vi "compute_average_movie.vi"(8 "error in (no error)":errorcluster, 10 "movies":refnum<class "ImageCollection.lvclass">[](array[class])) -> (0 "error out":errorcluster, 2 "average movie":refnum<class "ImageCollection.lvclass">)   [LabVIEW 2010, in "ImageCollection.lvclass"]
uses:
  ImageCollection.lvclass
  Image/Image/Image.lvclass
  add_mode_enum.ctl
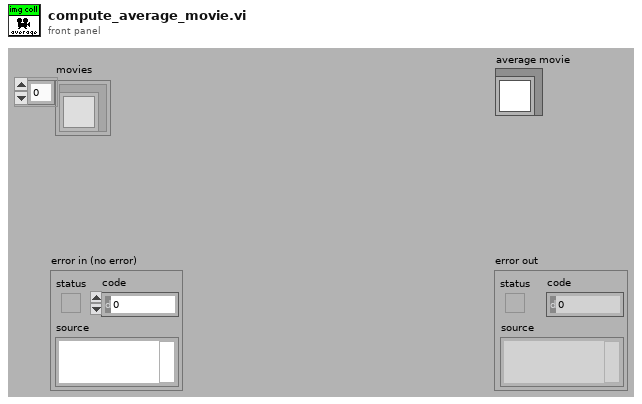
[diagram p1: front panel]
types:
  T1 = typedef "ImageCollection.lvclass/add_mode_enum.ctl" = enum16{"instance", "copy"}
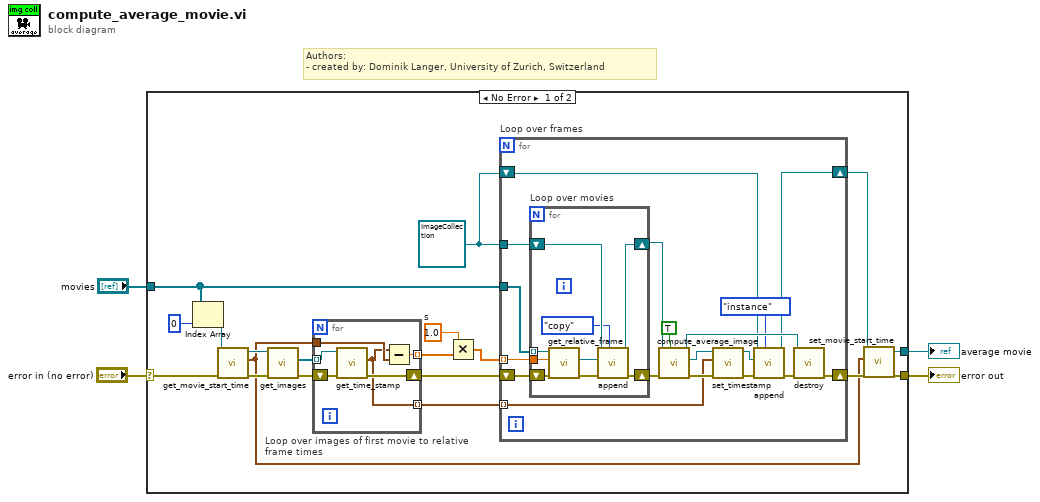
[diagram p0: block diagram]
diagram:
  # "Authors: \n- created by: Dominik Langer, University of Zurich, Switzerland"
  n1 = case shown="No Error" "error in (no error)" {
    selector: "error in (no error)" -> [w18 w57]
    tunnel: [w12 w57] -> w3
    tunnel: "movies" -> [w19 _]
    tunnel: [w10 _] -> w1
    frame No Error {
      w15 = refnum<class "ImageCollection.lvclass"> refnum ("ImageCollection.lvclass")
      w7 = dbl[unit] 1.0  # s
      n2 = Index Array(array=w19, index=0) -> (element=w16:refnum<class "ImageCollection.lvclass">)
      n3 = call-dynamic "get_movie_start_time.vi"("error in (no error)"=w18, "ImageCollection.lvclass in"=w16) -> ("error out"=w17:errorcluster, "movie start"=w9:timestamp, "ImageCollection.lvclass out"=w14:refnum<class "ImageCollection.lvclass">)  [unwired: 7 out]
      n4 = call-dynamic "get_images.vi"("error in (no error)"=w17, "ImageCollection.lvclass in"=w14) -> ("error out"=w23:errorcluster, "images"=w21:refnum<class "Image.lvclass">[])  [unwired: 8 out]
      n5 = for "Loop over images of first movie to relative frame times" {
        tunnel: w21 -> [w55] mode=indexing
        shift-right: [w54] -> w20
        shift-left: w23 -> [w56]
        tunnel: w9 -> [w53]
        tunnel: [w52] -> w6 mode=indexing
        tunnel: [w51] -> w8 mode=indexing
        n6 = call-dynamic "get_time_stamp.vi"("error in (no error)"=w56, "Image.lvclass in"=w55) -> ("error out"=w54:errorcluster, "timestamp"=w51:timestamp)  [unwired: 8 out]
        n7 = Subtract(x=w51, y=w53) -> (x-y=w52:dbl)
      }
      n8 = Multiply(x=w7, y=w6) -> (x*y=w5:dbl[unit][])
      n9 = for "Loop over frames" {
        shift-right: [w33] -> w13
        shift-left: w20 -> [w41]
        tunnel: w19 -> [w39]
        tunnel: w15 -> [w38]
        shift-right: [w29] -> w11
        shift-left: w15 -> [w32]
        tunnel: w5 -> [w40] mode=indexing
        tunnel: w8 -> [w25] mode=indexing
        n10 = for "Loop over movies" {
          tunnel: w40 -> [w49]
          tunnel: w39 -> [w48] mode=indexing
          shift-right: [w47] -> w37
          shift-left: w41 -> [w50]
          shift-right: [w44] -> w36
          shift-left: w38 -> [w46]
          n11 = call-dynamic "get_relative_frame.vi"("error in (no error)"=w50, "relative time"=w49, "ImageCollection in"=w48) -> ("error out"=w43:errorcluster, "frame"=w42:refnum<class "Image.lvclass">)  [unwired: 1 in, 6 out]
          n12 = call-dynamic "append.vi"("add mode"=add_mode_enum."copy", "error in (no error)"=w43, "Image.lvclass"=w42, "ImageCollection in"=w46) -> ("error out"=w47:errorcluster, "ImageCollection out"=w44:refnum<class "ImageCollection.lvclass">)  [unwired: 6 out]
        }
        n13 = call-dynamic "compute_average_image.vi"("all?"=TRUE, "error in (no error)"=w37, "ImageCollection in"=w36) -> ("error out"=w28:errorcluster, "averaged image"=w27:refnum<class "Image.lvclass">, "ImageCollection out"=w34:refnum<class "ImageCollection.lvclass">)  [unwired: 2 in, 4 out]
        n14 = call-dynamic "set_timestamp.vi"("error in (no error)"=w28, "timestamp"=w25, "Image.lvclass in"=w27) -> ("error out"=w26:errorcluster, "Image.lvclass out"=w24:refnum<class "Image.lvclass">)  [unwired: 7 out]
        n15 = call-dynamic "append.vi"("add mode"=add_mode_enum."instance", "error in (no error)"=w26, "Image.lvclass"=w24, "ImageCollection in"=w32) -> ("error out"=w30:errorcluster, "ImageCollection out"=w29:refnum<class "ImageCollection.lvclass">)  [unwired: 6 out]
        n16 = call-dynamic "destroy.vi"("error in (no error)"=w30, "ImageCollection in"=w34) -> ("error out"=w33:errorcluster)  [unwired: 9 out]
      }
      n17 = call-dynamic "set_movie_start_time.vi"("error in (no error)"=w13, "movie start"=w9, "ImageCollection.lvclass in"=w11) -> ("error out"=w12:errorcluster, "ImageCollection.lvclass out"=w10:refnum<class "ImageCollection.lvclass">)  [unwired: 7 out]
    }
    frame Error {
    }
  }
  "error out" <- w3
  "average movie" <- w1
